vi "Configure Constant Current.vi"(8 "error in (no error)":errorcluster, 10 "CC Current (0)":dbl min=0.0 max=240.0 step=1.0 format="%#.4f", 11 "VISA resource name":refnum<visa-resource-name>) -> (0 "error out":errorcluster, 3 "VISA resource name out":refnum<visa-resource-name>)   [LabVIEW 2024, in "BK Precision 8500B Series.lvlib"]
doc: "Configures the current and voltage max/min limits for constant current (CC) operation."
uses:
  BK Precision 8500B Series.lvlib
panel:
  # "A"
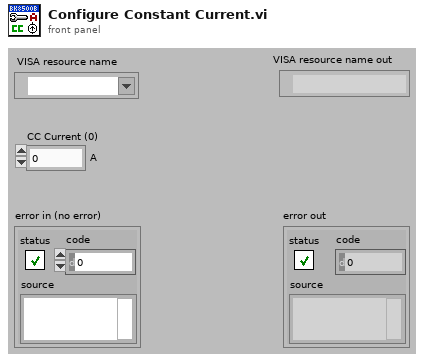
[diagram p1: front panel]
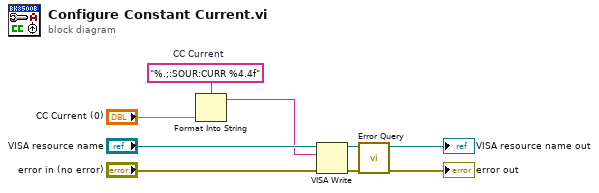
[diagram p0: block diagram]
diagram:
  w7 = "%.;:SOUR:CURR %4.4f"  # CC Current
  n1 = Format Into String(format string=w7, "CC Current (0)") -> (resulting string=w1:string)  [unwired: 2 in, 1 out]
  n2 = VISA Write(VISA resource name="VISA resource name", write buffer=w1, error in (no error)="error in (no error)") -> (VISA resource name out=w5:refnum<visa-resource-name>, error out=w6:errorcluster)  [unwired: 1 out]
  n3 = call "Error Query.vi"("error in (no error)"=w6, "VISA resource name"=w5) -> ("error out"=→"error out":errorcluster, "VISA resource name out"=→"VISA resource name out":refnum<visa-resource-name>)  [unwired: 6 in, 2 out]
